vi "Examen.vi"() -> ()   [LabVIEW 2010]
panel:
  out "CAMBIO":dbl
  in  "$25":bool
  in  "$35":bool
  in  "$18":bool
  out "?":string
  in  "DINERO":dbl
  out "?":dbl(slide) scale=0.0..100.0
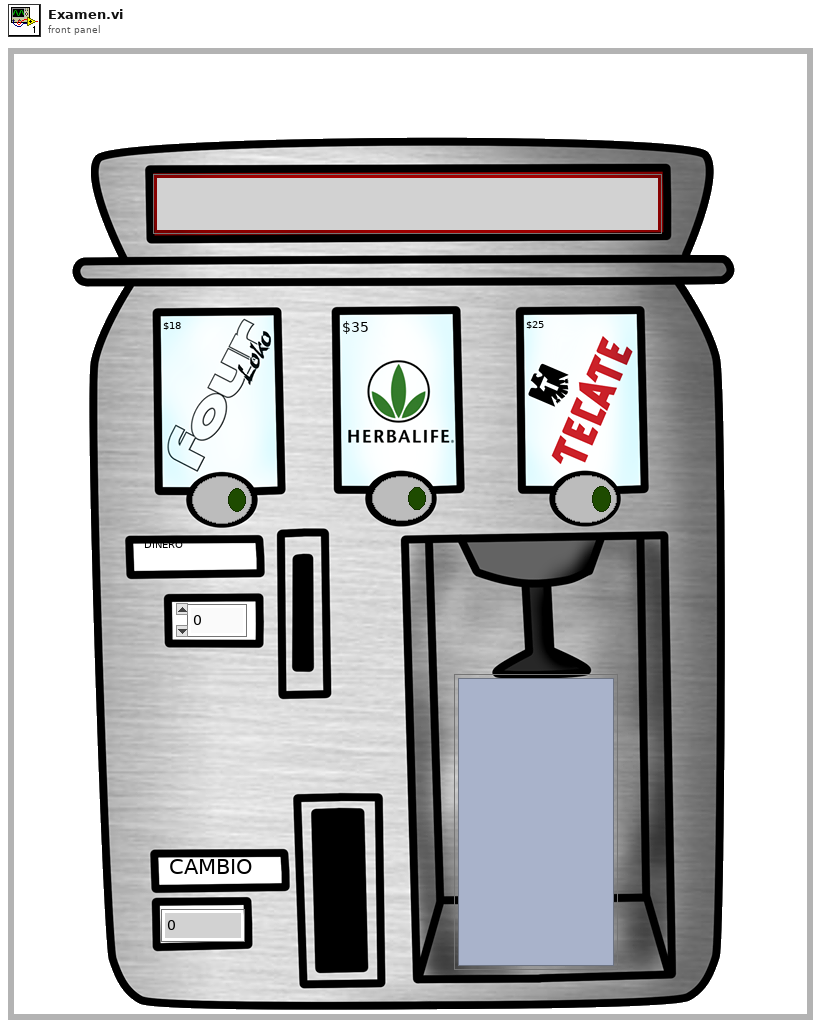
[diagram p1: front panel]
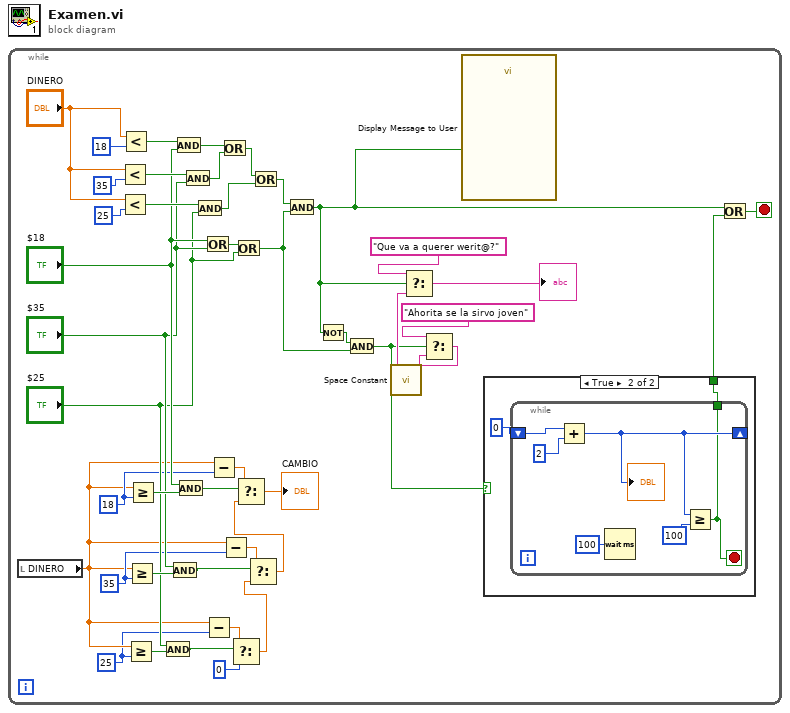
[diagram p0: block diagram]
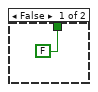
[diagram p2: hidden frame]
diagram:
  n1 = while {
    stop <- w3 stop-if-true
    w7 = 25
    w12 = 35
    w15 = 18
    n2 = local read "DINERO"() -> (w8:dbl)
    n3 = Less?(x="DINERO", y=35) -> (x < y?=w39:bool)
    n4 = Less?(x="DINERO", y=25) -> (x < y?=w38:bool)
    n5 = Less?(x="DINERO", y=18) -> (x < y?=w40:bool)
    n6 = Greater Or Equal?(x=w8, y=w7) -> (x >= y?=w19:bool)
    n7 = Greater Or Equal?(x=w8, y=w12) -> (x >= y?=w21:bool)
    n8 = Greater Or Equal?(x=w8, y=w15) -> (x >= y?=w23:bool)
    n9 = And(x="$25", y=w19) -> (x .and. y?=w11:bool)
    n10 = And(x="$35", y=w21) -> (x .and. y?=w14:bool)
    n11 = And(x=w40, y="$18") -> (x .and. y?=w37:bool)
    n12 = And(x="$18", y=w23) -> (x .and. y?=w17:bool)
    n13 = And(x=w39, y="$35") -> (x .and. y?=w36:bool)
    n14 = And(x=w38, y="$25") -> (x .and. y?=w35:bool)
    n15 = Or(x="$18", y="$35") -> (x .or. y?=w33:bool)
    n16 = Subtract(x=w8, y=w7) -> (x-y=w10:dbl)
    n17 = Subtract(x=w8, y=w15) -> (x-y=w16:dbl)
    n18 = Or(x=w37, y=w36) -> (x .or. y?=w34:bool)
    n19 = Subtract(x=w8, y=w12) -> (x-y=w13:dbl)
    n20 = Select(t=w10, s=w11, f=0) -> (s? t:f=w5:dbl)
    n21 = Or(x=w33, y="$25") -> (x .or. y?=w29:bool)
    n22 = Select(t=w13, s=w14, f=w5) -> (s? t:f=w6:dbl)
    n23 = Select(t=w16, s=w17, f=w6) -> (s? t:f=→"CAMBIO":dbl)
    n24 = Or(x=w34, y=w35) -> (x .or. y?=w32:bool)
    n25 = And(x=w32, y=w29) -> (x .and. y?=w2:bool)
    n26 = Not(x=w2) -> (.not. x?=w26:bool)
    n27 = And(x=w26, y=w29) -> (x .and. y?=w25:bool)
    n28 = call <vilib>:"Space Constant.vi"() -> ("String"=w24:string)
    n29 = Select(t="Ahorita se la sirvo joven", s=w25, f=w24) -> (s? t:f=w28:string)
    n30 = Select(t="Que va a querer werit@?", s=w2, f=w28) -> (s? t:f=→"?":string)
    n31 = call "Display Message to User"("Enable"=w2) -> ()  [unwired: 9 in, 2 out]
    n32 = case shown="True" w25 {
      tunnel: [FALSE w46] -> w1
      frame False {
      }
      frame True {
        n33 = while {
          shift-right: [w49] -> _
          shift-left: 0 -> [w53]
          tunnel: [w48] -> w46
          stop <- w48 stop-if-true
          n34 = Add(x=w53, y=2) -> (x+y=w49:i32)
          "?" <- w49
          n35 = Wait (ms)(milliseconds to wait=100) -> ()  [unwired: 1 out]
          n36 = Greater Or Equal?(x=w49, y=100) -> (x >= y?=w48:bool)
        }
      }
    }
    n37 = Or(x=w2, y=w1) -> (x .or. y?=w3:bool)
  }
